vi "Query Active DUT Audio Call Action State.vi"(8 "error in (no error)":errorcluster, 10 "SIM Slot (1)":i32=1, 11 "VISA resource name":refnum<visa-resource-name>) -> (0 "error out":errorcluster, 1 "Disconnect":i32, 2 "Connect":i32, 3 "VISA resource name out":refnum<visa-resource-name>, 4 "Accept":i32, 5 "Reject":i32)   [LabVIEW 2015, in "Rohde&Schwarz CMXP Base.lvlib"]
doc: "Queries the states of audio call actions.\n\nAttribute:\nRSCMXPBASE_ATTR_SELECT_ACTIVE_DUT_SIM_SLOT\n\nRemote-control command:\nFETCh:DUT:MODem<ModemIdx>:CONTrol:CALL:AUDio:STATe?"
uses:
  <instrlib>/Rohde&Schwarz CMXP Base/Rohde&Schwarz CMXP Base.lvlib
  <instrlib>/Rohde&Schwarz CMXP Base/Private/rsidr_core.llb/rsidr_core.lvlib
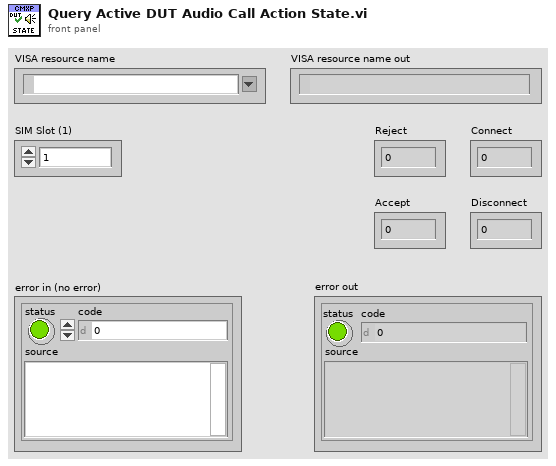
[diagram p1: front panel]
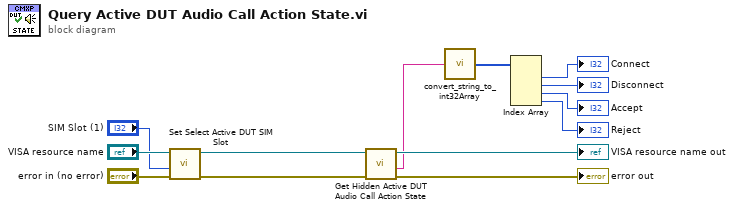
[diagram p0: block diagram]
diagram:
  n1 = call "Set Select Active DUT SIM Slot"("error in (no error)"="error in (no error)", "Select Active DUT SIM Slot (0)"="SIM Slot (1)", "instrument handle"="VISA resource name") -> ("error out"=w10:errorcluster, "instrument handle out"=w11:refnum<visa-resource-name>)  [unwired: 7 in]
  n2 = call "Get Hidden Active DUT Audio Call Action State"("error in (no error)"=w10, "instrument handle"=w11) -> ("error out"=→"error out":errorcluster, "Hidden Active DUT Audio Call Action State"=w5:string, "instrument handle out"=→"VISA resource name out":refnum<visa-resource-name>)  [unwired: 7 in]
  n3 = call <instrlib>:"convert_string_to_int32Array.vi"("string in"=w5) -> ("int32 array out"=w9:i32[])  [unwired: 3 in, 1 out]
  n4 = Index Array(array=w9) -> (element #1=→"Connect":i32, element #2=→"Disconnect":i32, element #3=→"Accept":i32, element #4=→"Reject":i32)  [unwired: 4 in]
